vi "Test Method Details.vi"(8 "error in (no error)":errorcluster, 10 "vi path":path) -> (0 "error out":errorcluster, 1 "Test Case Class":string, 2 "Test Method":string, 4 "Test Case Path":path)   [LabVIEW 2020, in "Execution UI.lvclass"]
uses:
  Execution UI.lvclass
  LUnit Test Case.lvclass
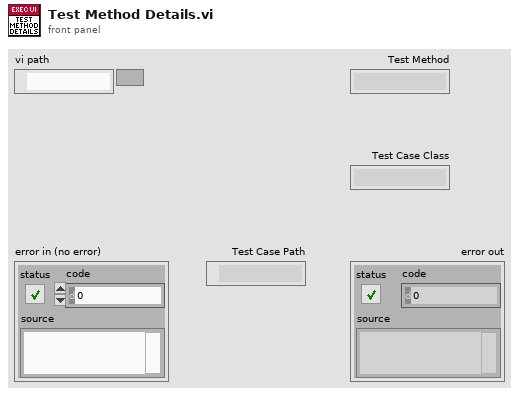
[diagram p1: front panel]
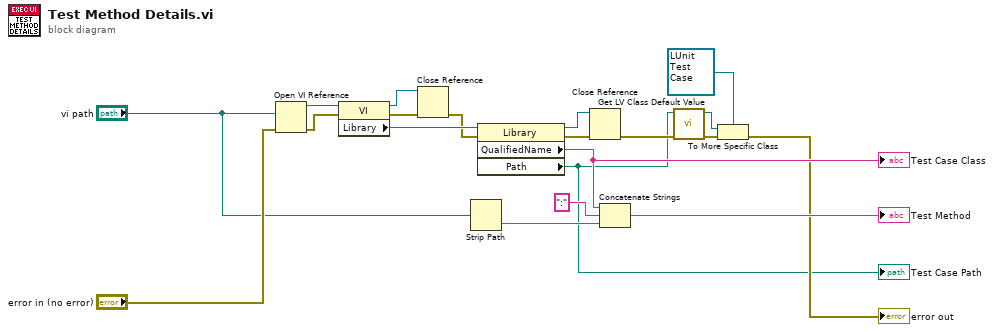
[diagram p0: block diagram]
diagram:
  n1 = Open VI Reference(vi path="vi path", error in (no error)="error in (no error)") -> (vi reference=w20:refnum<vi>, error out=w19:errorcluster)  [unwired: 4 in]
  n2 = property class="VI"(reference=w20, error in=w19) -> (reference out=w14:refnum<vi>, error out=w16:errorcluster, "Library"=w18:refnum<vi>)
  n3 = Close Reference(reference=w14, error in (no error)=w16) -> (error out=w15:errorcluster)
  n4 = Strip Path(path="vi path") -> (name=w9:string)  [unwired: 1 out]
  n5 = property class="Library"(reference=w18, error in=w15) -> (reference out=w13:refnum<vi>, error out=w17:errorcluster, "QualifiedName"=w11:string, "Path"=w3:path)
  "Test Case Class" <- w11
  "Test Case Path" <- w3
  n6 = Close Reference(reference=w13, error in (no error)=w17) -> (error out=w8:errorcluster)
  n7 = Concatenate Strings(w11, ":" ("string"), w9) -> (→"Test Method":string)
  n8 = call <vilib>:"Get LV Class Default Value.vi"("error in (no error)"=w8, "class path"=w3) -> ("error out"=w4:errorcluster, "object"=w2:refnum<class>)  [unwired: 8 in]
  n9 = To More Specific Class(target class=refnum<class "LUnit Test Case.lvclass"> refnum ("LUnit Test Case.lvclass"), reference=w2, error in=w4) -> (error out=→"error out":errorcluster)  [unwired: 1 out]
